vi "Auton move distance.vi"(0 "Distance":dbl=3.0 format="%#_13g", 1 "PID gains":T1 {"derivative time (Td, min)" format="%.3f"; "integral time (Ti, min)" format="%.3f"; "proportional gain (Kc)" format="%.3f"}, 2 "PID Complete Delay":u32, 3 "Refnum in":refnum<k33>) -> (7 "Distance Travelled":dbl, 10 "rt fifo out":refnum<k33>)   [LabVIEW 2014]
uses:
  TeleopCmd.ctl
  CmdFlag.ctl
  AutonCals.vi
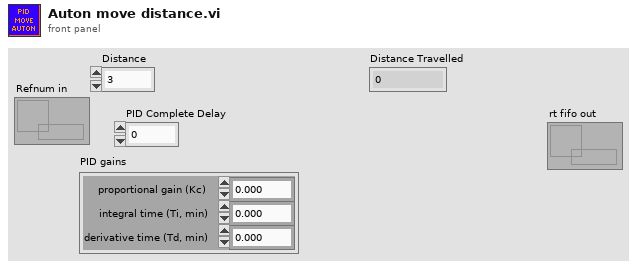
[diagram p1: front panel]
types:
  T1 = cluster{"proportional gain (Kc)":dbl, "integral time (Ti, min)":dbl, "derivative time (Td, min)":dbl}
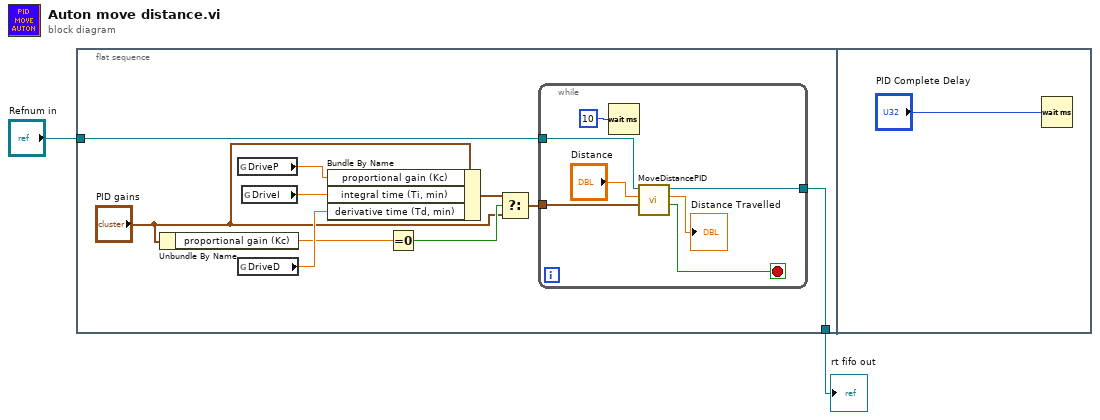
[diagram p0: block diagram]
diagram:
  n1 = flat-sequence {
    tunnel: "Refnum in" -> [w12]
    tunnel: [w3] -> w1
    frame #0 {
      n2 = Unbundle By Name("PID gains") -> ("proportional gain (Kc)"=w7:dbl)
      n3 = global read "AutonCals.vi" "DriveP"() -> (w9:dbl)
      n4 = global read "AutonCals.vi" "DriveD"() -> (w10:dbl)
      n5 = global read "AutonCals.vi" "DriveI"() -> (w11:dbl)
      n6 = Bundle By Name(cluster="PID gains", "proportional gain (Kc)"=w9, "integral time (Ti, min)"=w11, "derivative time (Td, min)"=w10) -> (w6:T1)
      n7 = Equal To 0?(x=w7) -> (x = 0?=w8:bool)
      n8 = Select(t=w6, s=w8, f="PID gains") -> (s? t:f=w4:T1)
      n9 = while {
        tunnel: w12 -> [w18]
        tunnel: w4 -> [w15]
        tunnel: [w14] -> w3
        stop <- w19 stop-if-true
        n10 = Wait (ms)(milliseconds to wait=u32 10) -> ()  [unwired: 1 out]
        n11 = call "MoveDistancePID.vi"("PID gains"=w15, "Distance"="Distance", "Refnum in"=w18) -> ("Boolean"=w19:bool, "Distance Travelled"=→"Distance Travelled":dbl, "Refnum out"=w14:refnum<k33>)  [unwired: 6 in]
      }
    }
    frame #1 {
      n12 = Wait (ms)(milliseconds to wait="PID Complete Delay") -> ()  [unwired: 1 out]
    }
  }
  "rt fifo out" <- w1
